vi "writeToXML.vi"(8 "error in (no error)":errorcluster, 10 "ClassLabel":string, 11 "GuiderMeasuredError in":refnum<class "GuiderMeasuredError.lvclass">) -> (0 "error out":errorcluster, 2 "XML out":string, 3 "GuiderMeasuredError out":refnum<class "GuiderMeasuredError.lvclass">)   [LabVIEW 2022 SP3, in "TCSDataDefinitions.lvlib" / "TCSGuiderCommand.lvlib" / "GuiderMeasuredError.lvclass"]
uses:
  GuiderMeasuredError.lvclass
  <userlib>/Common/UnitsAndXML/FlattenItemWithUnitToXML/FlattenLengthToXML/LengthUnit.ctl
  GuiderMeasuredError.lvclass/GuiderMeasuredError.ctl
  TCSGuiderCommand/TCSGuiderCommand.lvclass
  <userlib>/Common/UnitsAndXML/UnitsAndXML.lvlib
  <userlib>/Common/XML/XMLGenerator/XMLGenerator.lvclass
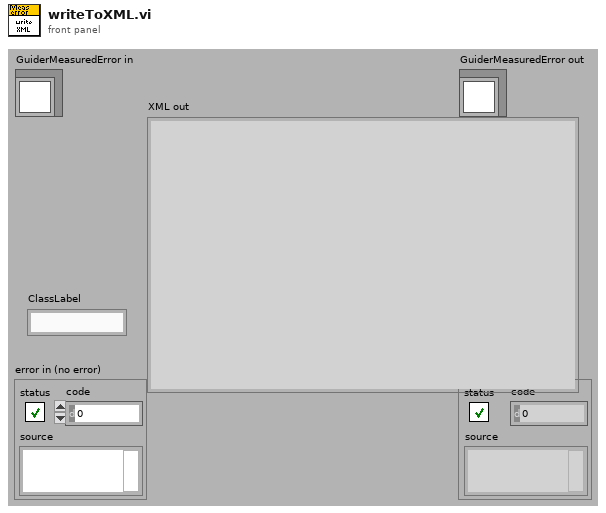
[diagram p1: front panel]
types:
  T1 = typedef "UnitsAndXML.lvlib/LengthUnit.ctl" = enum16{"m", "Angstrom", "AU", "chain", "cm", "cubit", "fathom", "fermi", "ft", "furlong", "hubble", "in", "ly", "mi", "mm", "rod", "um", "yd"}
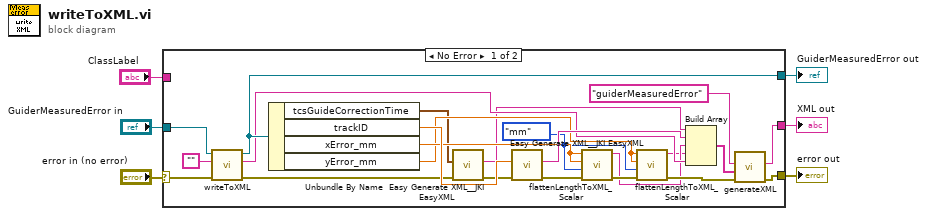
[diagram p0: block diagram]
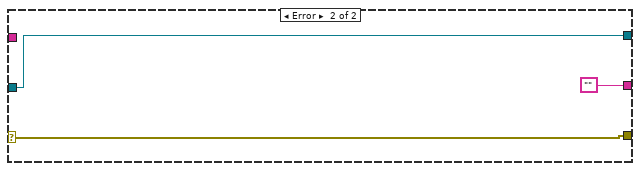
[diagram p2: hidden frame]
diagram:
  n1 = case shown="No Error" "error in (no error)" {
    selector: "error in (no error)" -> [w26 w32]
    tunnel: [w14 w32] -> w5
    tunnel: [w28 w31] -> w3
    tunnel: "GuiderMeasuredError in" -> [w29 w31]
    tunnel: [w15 ""] -> w2
    tunnel: "ClassLabel" -> [_ _]
    frame No Error {
      w22 = LengthUnit."mm" ("lengthUnitInXML")
      n2 = call-parent "writeToXML.vi"("error in (no error)"=w26, "ClassLAbel"="", "TCSGuiderCommand.lvclass"=w29) -> ("error out"=w10:errorcluster, "XML out"=w13:string, "TCSGuiderCommand.lvclass 2"=w28:refnum<class "GuiderMeasuredError.lvclass">)  [unwired: 6 in]
      n3 = Unbundle By Name(w28) -> ("tcsGuideCorrectionTime"=w8:timestamp, "trackID"=w25:dbl, "xError_mm"=w23:dbl[unit], "yError_mm"=w21:dbl[unit])
      n4 = call <vilib>:"Easy Generate XML__JKI EasyXML.vi"("error in (no error)"=w10, "LabVIEW Data"=w8) -> ("error out"=w9:errorcluster, "XML String"=w7:string)  [unwired: 8 in]
      n5 = call <vilib>:"Easy Generate XML__JKI EasyXML.vi"("error in (no error)"=w9, "LabVIEW Data"=w25) -> ("error out"=w19:errorcluster, "XML String"=w24:string)  [unwired: 8 in]
      n6 = call <userlib>:"flattenLengthToXML_Scalar.vi"("error in (no error)"=w19, "lengthUnitInXML"=w22, "lengthAgain"=w23, "length"=w23) -> ("error out"=w20:errorcluster, "xmlString"=w12:string)  [unwired: 6 in]
      n7 = call <userlib>:"flattenLengthToXML_Scalar.vi"("error in (no error)"=w20, "lengthUnitInXML"=w22, "lengthAgain"=w21, "length"=w21) -> ("error out"=w16:errorcluster, "xmlString"=w11:string)  [unwired: 6 in]
      n8 = Build Array(w7, w24, w12, w11, w13) -> (w18:string[])
      n9 = call <userlib>:"generateXML.vi"("error in"=w16, "childrenXML"=w18, "elementName"="guiderMeasuredError" ("Class Label")) -> ("error out"=w14:errorcluster, "XML out"=w15:string)  [unwired: 6 in, 1 out]
    }
    frame Error {
    }
  }
  "error out" <- w5
  "GuiderMeasuredError out" <- w3
  "XML out" <- w2
